vi "Result display event_UI.vi"(9 "Result Cluster":T5, 10 "Result cluster details":T3={"MNA"=[], "ISIM"=[], "Image update"=[{"Rack Id"=0, "Update image"=[TRUE, TRUE, FALSE, FALSE]}, {"Rack Id"=1, "Update image"=[FALSE, FALSE, TRUE, TRUE]}], "Current rack Id"=0, "LSL"=[], "USL"=[]}, 11 "InspectionCluster in":T4) -> (1 "output cluster":T2, 3 "InspectionCluster out":T4)   [LabVIEW 2019, in "ZenGage v3.0 UI.lvclass"]
uses:
  ZenGage v3.0 UI.lvclass
  <vilib>/vision/Image Controls.llb/IMAQ Image.ctl
  Type Definitions/Inspection/Result Cluster.ctl
  Type Definitions/Inspection/Inspection Cluster.ctl
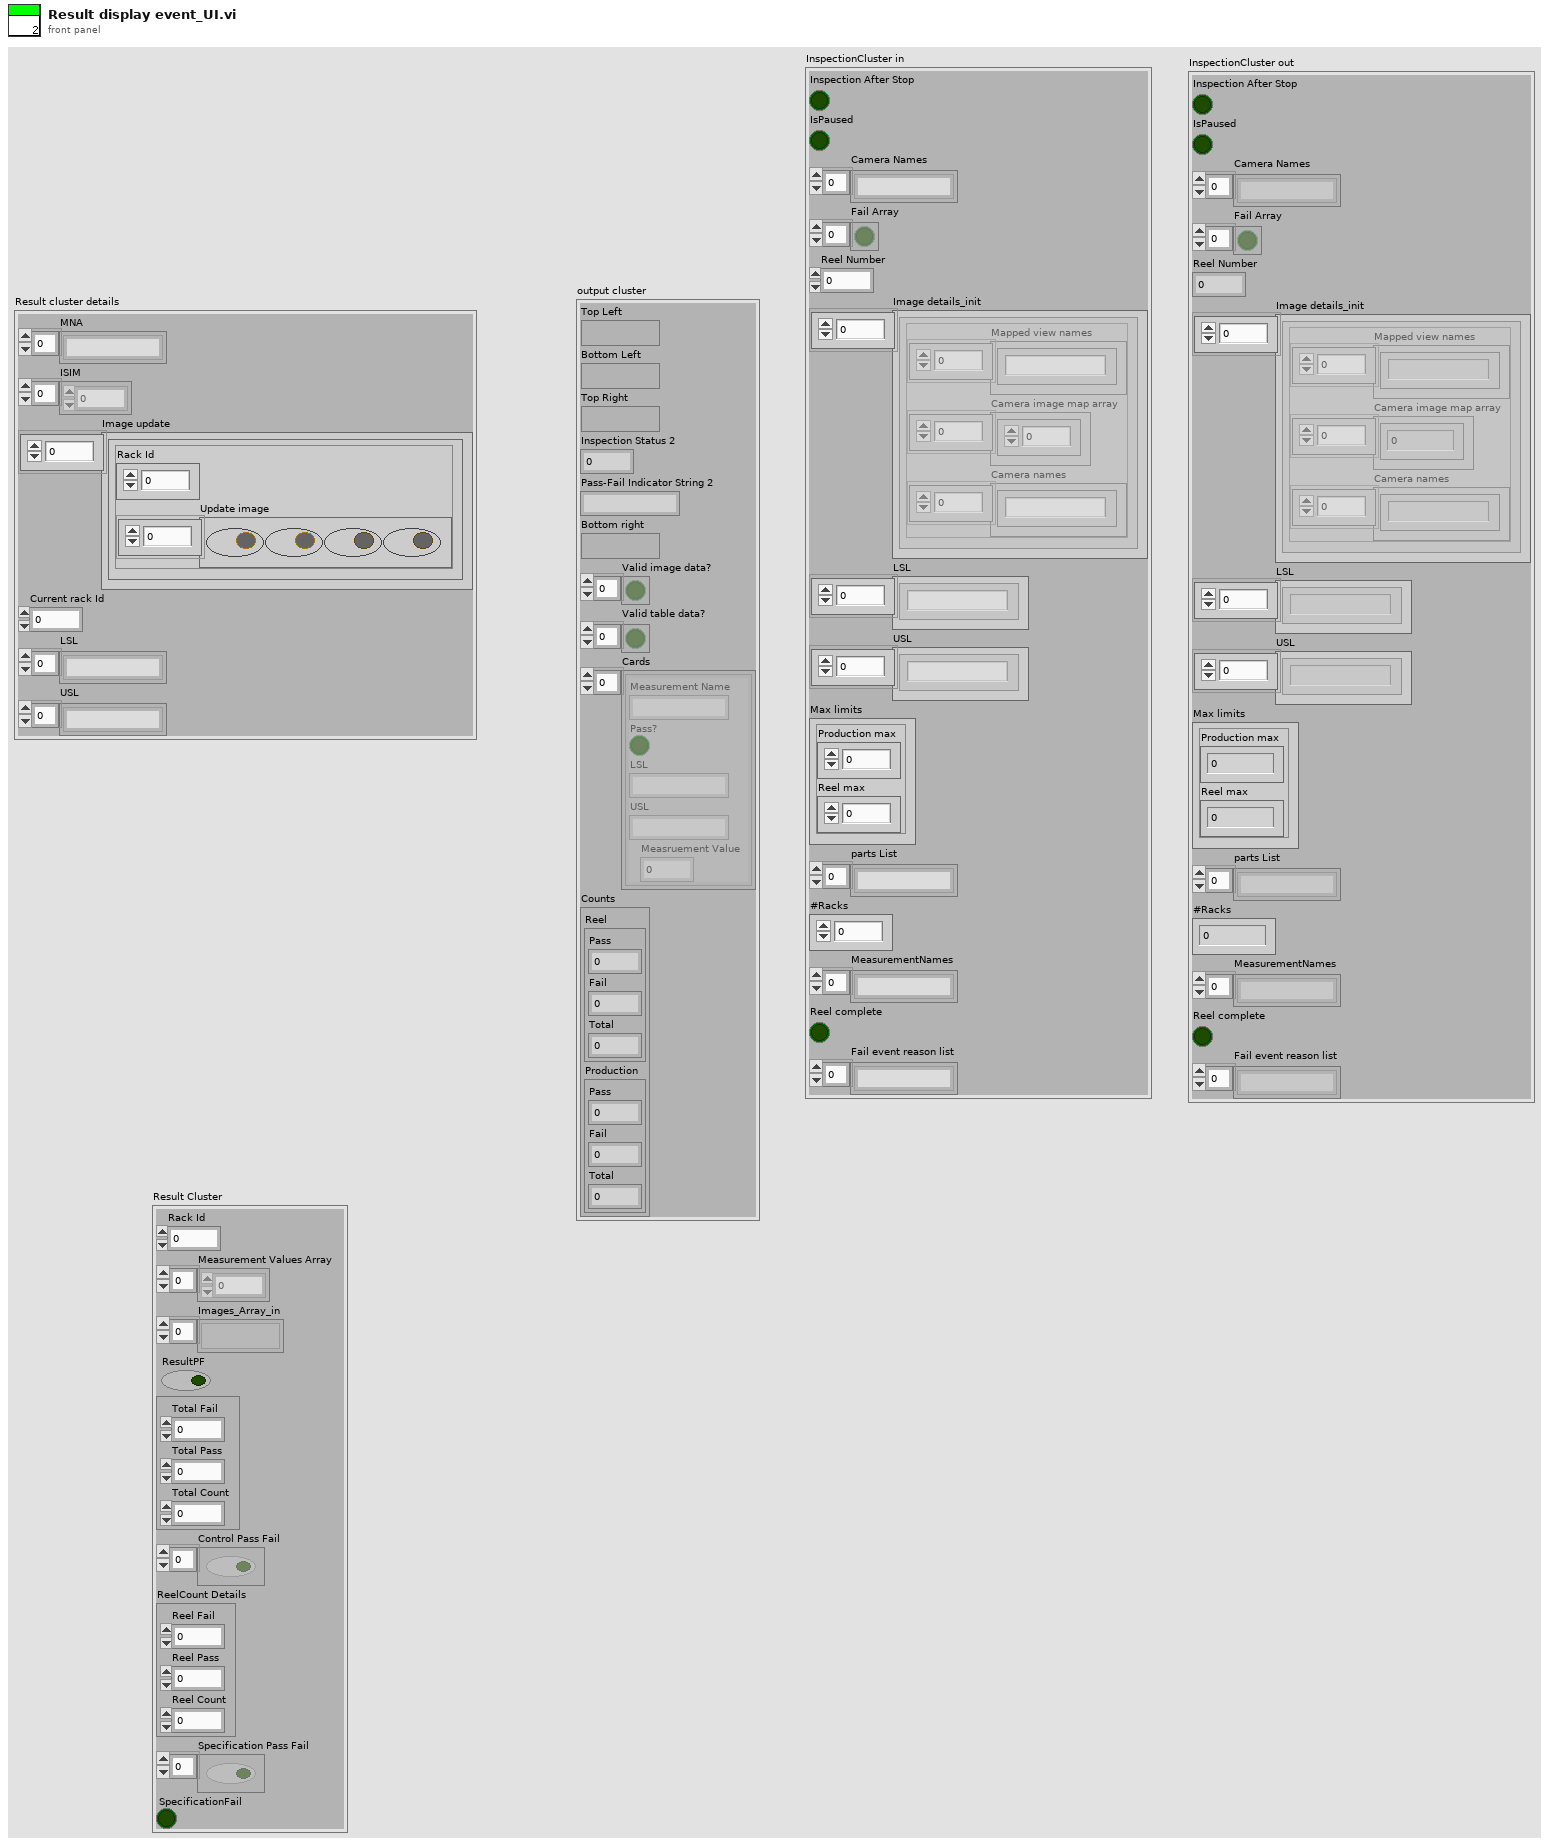
[diagram p1: front panel]
types:
  T1 = typedef "IMAQ Image.ctl" = refnum<image>
  T2 = cluster{"Top Left":T1, "Bottom Left":T1, "Top Right":T1, "Inspection Status 2":u32, "Pass-Fail Indicator String 2":string, "Bottom right":T1, "Valid image data?":bool[], "Valid table data?":bool[], "Cards":cluster{"Measurement Name":string, "Pass?":bool, "LSL":string, "USL":string, "Measruement Value":dbl}[], "Counts":cluster{"Reel":cluster{"Pass":u64, "Fail":u64, "Total":u64}, "Production":cluster{"Pass":u64, "Fail":u64, "Total":u64}}}
  T3 = cluster{"MNA":string[], "ISIM":u8[], "Image update":cluster{"Rack Id":i32, "Update image":bool[]}[], "Current rack Id":u8, "LSL":string[], "USL":string[]}
  T4 = typedef "ZenGage v3.0 UI.lvclass/Inspection Cluster.ctl" = cluster{"Inspection After Stop":bool, "IsPaused":bool, "Camera Names":string[], "Fail Array":bool[], "Reel Number":u32, "Image details_init":cluster{"Mapped view names":string[], "Camera image map array":i32[], "Camera names":string[]}[], "LSL":string[], "USL":string[], "Max limits":cluster{"Production max":u64, "Reel max":u64}, "parts List":string[], "#Racks":u8, "MeasurementNames":string[], "Reel complete":bool, "Fail event reason list":string[]}
  T5 = typedef "ZenGage v3.0 UI.lvclass/Result Cluster.ctl" = cluster{"Rack Id":u64, "Measurement Values Array ":dbl[], "Images_Array_in":T1[], "ResultPF":bool, "Production count details":cluster{"Total Count":dbl, "Total Pass":dbl, "Total Fail":dbl}, "Control Pass Fail":bool[], "ReelCount Details":cluster{"Reel Count":dbl, "Reel Pass":dbl, "Reel Fail":dbl}, "Specification Pass Fail":bool[], "SpecificationFail":bool}
  T6 = cluster{"Reel":cluster{"Pass":u64, "Fail":u64, "Total":u64}, "Production":cluster{"Pass":u64, "Fail":u64, "Total":u64}}
  T7 = cluster{"Total Count":dbl, "Total Pass":dbl, "Total Fail":dbl}
  T8 = cluster{"Reel Count":dbl, "Reel Pass":dbl, "Reel Fail":dbl}
  T9 = cluster{"Measurement Name":string, "Pass?":bool, "LSL":string, "USL":string, "Measruement Value":dbl}
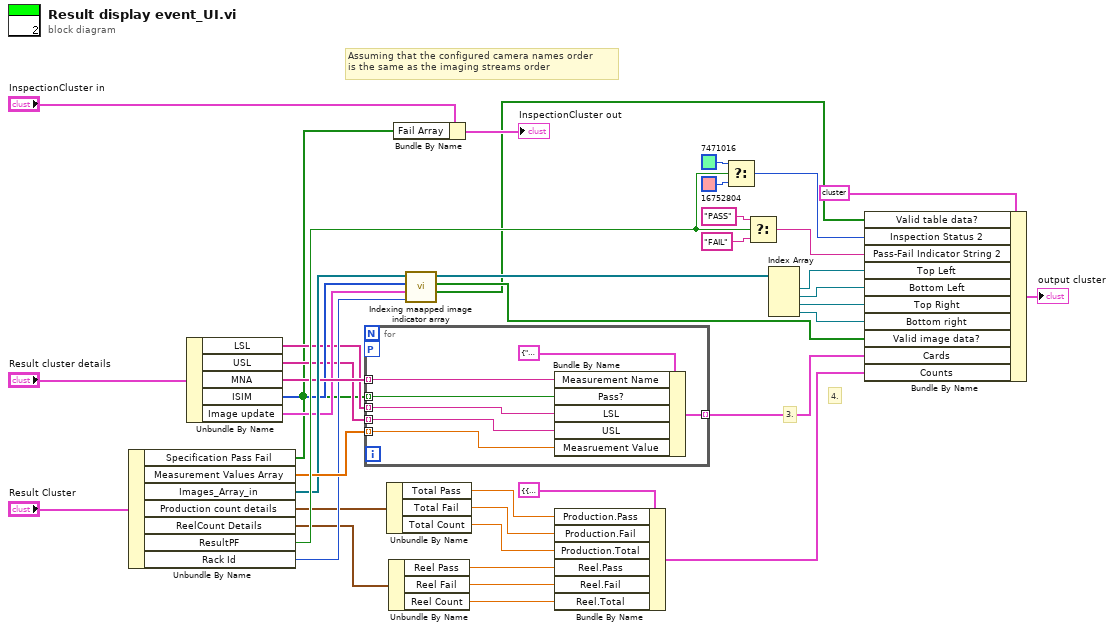
[diagram p0: block diagram]
diagram:
  # "4."
  # "3."
  # "Assuming that the configured camera names order\nis the same as the imaging streams order"
  n1 = Unbundle By Name("Result Cluster") -> ("Specification Pass Fail"=w1:bool[], "Measurement Values Array"=w39:dbl[], "Images_Array_in"=w35:T1[], "Production count details"=w27:T7, "ReelCount Details"=w26:T8, "ResultPF"=w40:bool, "Rack Id"=w30:u64)
  n2 = Unbundle By Name("Result cluster details") -> ("LSL"=w29:string[], "USL"=w28:string[], "MNA"=w33:string[], "ISIM"=w32:u8[], "Image update"=w31:cluster{"Rack Id":i32, "Update image":bool[]}[])
  n3 = for {
    tunnel: w39 -> [w41] mode=indexing
    tunnel: w33 -> [w47] mode=indexing
    tunnel: w1 -> [w46] mode=indexing
    tunnel: w29 -> [w44] mode=indexing
    tunnel: w28 -> [w43] mode=indexing
    tunnel: [w42] -> w12 mode=indexing
    workers-P: _ -> [_]
    n4 = Bundle By Name(cluster=T9 {"Measurement Name"="", "Pass?"=FALSE, "LSL"="", "USL"="", "Measruement Value"=0.0} ("Cluster"), "Measurement Name"=w47, "Pass?"=w46, "LSL"=w44, "USL"=w43, "Measruement Value"=w41) -> (w42:T9)
  }
  n5 = Unbundle By Name(w27) -> ("Total Pass"=w9:dbl, "Total Fail"=w8:dbl, "Total Count"=w7:dbl)
  n6 = Unbundle By Name(w26) -> ("Reel Pass"=w6:dbl, "Reel Fail"=w5:dbl, "Reel Count"=w4:dbl)
  n7 = Bundle By Name(cluster="InspectionCluster in", "Fail Array"=w1) -> (→"InspectionCluster out":T4)
  n8 = call "Indexing maapped image indicator array.vi"("Rack Id"=w30, "Image update"=w31, "ISIM"=w32, "Image array"=w35) -> ("Table update"=w13:bool[], "Update image"=w14:bool[], "mapped image arr out"=w16:T1[])  [unwired: 5 in]
  n9 = Bundle By Name(cluster=T6 {"Reel"={"Pass"=0, "Fail"=0, "Total"=0}, "Production"={"Pass"=0, "Fail"=0, "Total"=0}} ("Counts"), "Production.Pass"=w9, "Production.Fail"=w8, "Production.Total"=w7, "Reel.Pass"=w6, "Reel.Fail"=w5, "Reel.Total"=w4) -> (w10:T6)
  n10 = Select(t=u32 7471016, s=w40, f=u32 16752804) -> (s? t:f=w21:u32)
  n11 = Select(t="PASS", s=w40, f="FAIL") -> (s? t:f=w20:string)
  n12 = Index Array(array=w16) -> (element #1=w19:T1, element #2=w18:T1, element #3=w17:T1, element #4=w15:T1)  [unwired: 4 in]
  n13 = Bundle By Name(cluster=T2 {"Top Left"=refnum, "Bottom Left"=refnum, "Top Right"=refnum, "Inspection Status 2"=0, "Pass-Fail Indicator String 2"="", "Bottom right"=refnum, "Valid image data?"=[], "Valid table data?"=[], "Cards"=[], "Counts"={"Reel"={"Pass"=0, "Fail"=0, "Total"=0}, "Production"={"Pass"=0, "Fail"=0, "Total"=0}}} ("output cluster"), "Valid table data?"=w13, "Inspection Status 2"=w21, "Pass-Fail Indicator String 2"=w20, "Top Left"=w19, "Bottom Left"=w18, "Top Right"=w17, "Bottom right"=w15, "Valid image data?"=w14, "Cards"=w12, "Counts"=w10) -> (→"output cluster":T2)
